vi "Begin.vi"(11 "Image Size":T1=enum."160x120") -> (0 "error out":errorcluster)   [LabVIEW 2012]
doc: "Called before other user functions, this VI is expected to open initial I/O refnums, load in file data, and do all program initialization. Notice that the <B>error out</B> terminal is simply used for data flow. Wiring it to other structures or subVIs ensures that this VI runs first."
uses:
  <vilib>/Rock Robotics/WPI/Camera/WPI_CameraImageSize.ctl
  <vilib>/Rock Robotics/WPI/Camera/WPI_CameraWhite Balance Values.ctl
  <vilib>/Rock Robotics/WPI/Camera/WPI_CameraExposure Values.ctl
  <vilib>/Rock Robotics/WPI/Camera/WPI_CameraFrameRate.ctl
  <vilib>/Rock Robotics/WPI/DriverStation/WPI_DriverStationRobotMode2.ctl
  <vilib>/Rock Robotics/SystemInterfaces/DIO/FPGA_DIOPWMChannel.ctl
  <vilib>/Rock Robotics/WPI/Joystick/WPI_JoystickDeviceEnum.ctl
  <vilib>/Rock Robotics/SystemInterfaces/DIO/FPGA_DIOChannel.ctl
  <vilib>/Rock Robotics/SystemInterfaces/AI/FPGA_AIGyroChannel.ctl
  <vilib>/Rock Robotics/WPI/Relay/WPI_RelayDirection.ctl
  <vilib>/Rock Robotics/SystemInterfaces/DIO/FPGA_DIORelayChannel.ctl
  <vilib>/Rock Robotics/SystemInterfaces/Typedef/FPGA_TypedefDigitalModule.ctl
  <vilib>/Rock Robotics/SystemInterfaces/AI/FPGA_AIChannel.ctl
  Robot Global Data.vi
  <vilib>/Rock Robotics/WPI/MotorControl/WPI_MotorControlOpen Victor.vi
  <vilib>/Rock Robotics/WPI/MotorControl/WPI_MotorControlOpen Jaguar.vi
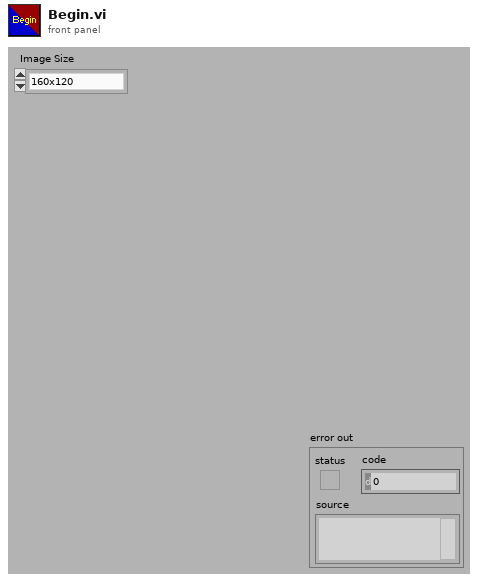
[diagram p1: front panel]
types:
  T1 = typedef "WPI_CameraImageSize.ctl" = enum16{"640x480", "320x240", "160x120"}
  T2 = typedef "FPGA_AIChannel.ctl" = enum8{"AI 1", "AI 2", "AI 3", "AI 4", "AI 5", "AI 6", "AI 7", "AI 8", "Invalid"}
  T3 = typedef "FPGA_DIOChannel.ctl" = enum8{"DIO 1", "DIO 2", "DIO 3", "DIO 4", "DIO 5", "DIO 6", "DIO 7", "DIO 8", "DIO 9", "DIO 10", "DIO 11", "DIO 12", "DIO 13", "DIO 14", "Invalid"}
  T4 = typedef "FPGA_TypedefDigitalModule.ctl" = enum16{"Digital Module 1", "Digital Module 2"}
  T5 = typedef "FPGA_DIOPWMChannel.ctl" = enum8{"PWM 1", "PWM 2", "PWM 3", "PWM 4", "PWM 5", "PWM 6", "PWM 7", "PWM 8", "PWM 9", "PWM 10", "Invalid"}
  T6 = typedef "FPGA_DIORelayChannel.ctl" = enum8{"Relay 1", "Relay 2", "Relay 3", "Relay 4", "Relay 5", "Relay 6", "Relay 7", "Relay 8", "Invalid"}
  T7 = typedef "WPI_RelayDirection.ctl" = enum16{"Both directions", "Forward only", "Reverse only"}
  T8 = typedef "FPGA_AIGyroChannel.ctl" = enum8{"AI 1", "AI 2", "Invalid"}
  T9 = typedef "WPI_JoystickDeviceEnum.ctl" = enum16{"USB 1", "USB 2", "USB 3", "USB 4", "Kinect 1", "Kinect 2"}
  T10 = typedef "WPI_DriverStationRobotMode2.ctl" = enum16{"Autonomous Disabled", "Autonomous Enabled", "Teleop Disabled", "Teleop Enabled", "Timeout", "Finish", "Test Disabled", "Test Enabled"}
  T11 = typedef "WPI_CameraFrameRate.ctl" = u32
  T12 = typedef "WPI_CameraExposure Values.ctl" = enum16{"Auto", "Flicker-free 50 Hz", "Flicker-free 60 Hz", "Hold current"}
  T13 = typedef "WPI_CameraWhite Balance Values.ctl" = enum16{"Auto", "Fixed indoor", "Fixed outdoor 1", "Fixed outdoor 2", "Fixed fluorescent 1", "Fixed fluorescent 2", "Hold current"}
  T14 = typedef "WPI_RelayDevRef.ctl" = cluster{"DevStatus":errorcluster, "Relay Channel":T6, "Digital Module":T4, "Relay Direction":T7}
  T15 = typedef "WPI_AnalogChannelDevRef.ctl" = cluster{"DevStatus":errorcluster, "Analog Module":T16, "Analog Channel":T2}
  T16 = typedef "FPGA_TypedefAnalogModule.ctl" = enum16{"Analog Module 1", "Analog Module 2"}
  T17 = typedef "WPI_DigitalInputDevRef.ctl" = cluster{"DevStatus":errorcluster, "DIO Channel":T3, "Digital Module":T4}
  T18 = typedef "WPI_CameraDevRef.ctl" = cluster{"Camera Address":string, "CameraStatus":errorcluster, "Acquire Image Notifier":refnum<notifier>}
  T19 = typedef "WPI_ServoDeviceRef.ctl" = cluster{"DeviceStatus":errorcluster, "Digital Module":T4, "PWM Channel":T5, "DeadBand":T20}
  T20 = typedef "WPI_PWMDeadband.ctl" = cluster{"Name":string, "maxPositivePwm":i32, "minPositivePwm":i32, "centerPwm":i32, "maxNegativePwm":i32, "minNegativePwm":i32, "angularRange":u16}
  T21 = typedef "WPI_MotorControlDeviceRef.ctl" = cluster{"DeviceStatus":errorcluster, "Type":enum16{"PWM", "CAN"}, "PWM":cluster{"Digital Module":T4, "PWM Channel":T5, "DeadBand":T20}, "CAN":cluster{"Device Number":u8, "Control Mode":T22, "Semaphore":T23, "Max Vout":dbl}, "Invert":bool, "TransformRef":T24, "InvTransformRef":T24}
  T22 = typedef "WPI_CANJaguar_ControlMode.ctl" = enum8{"Percent VBus", "Current", "Speed", "Position", "Voltage"}
  T23 = typedef "Semaphore RefNum" = refnum<k1>
  T24 = typedef "WPI_PWMTransform_ConPane.ctl" = refnum<vi>
  T25 = typedef "WPI_JoystickDevRef.ctl" = cluster{"Device":T9}
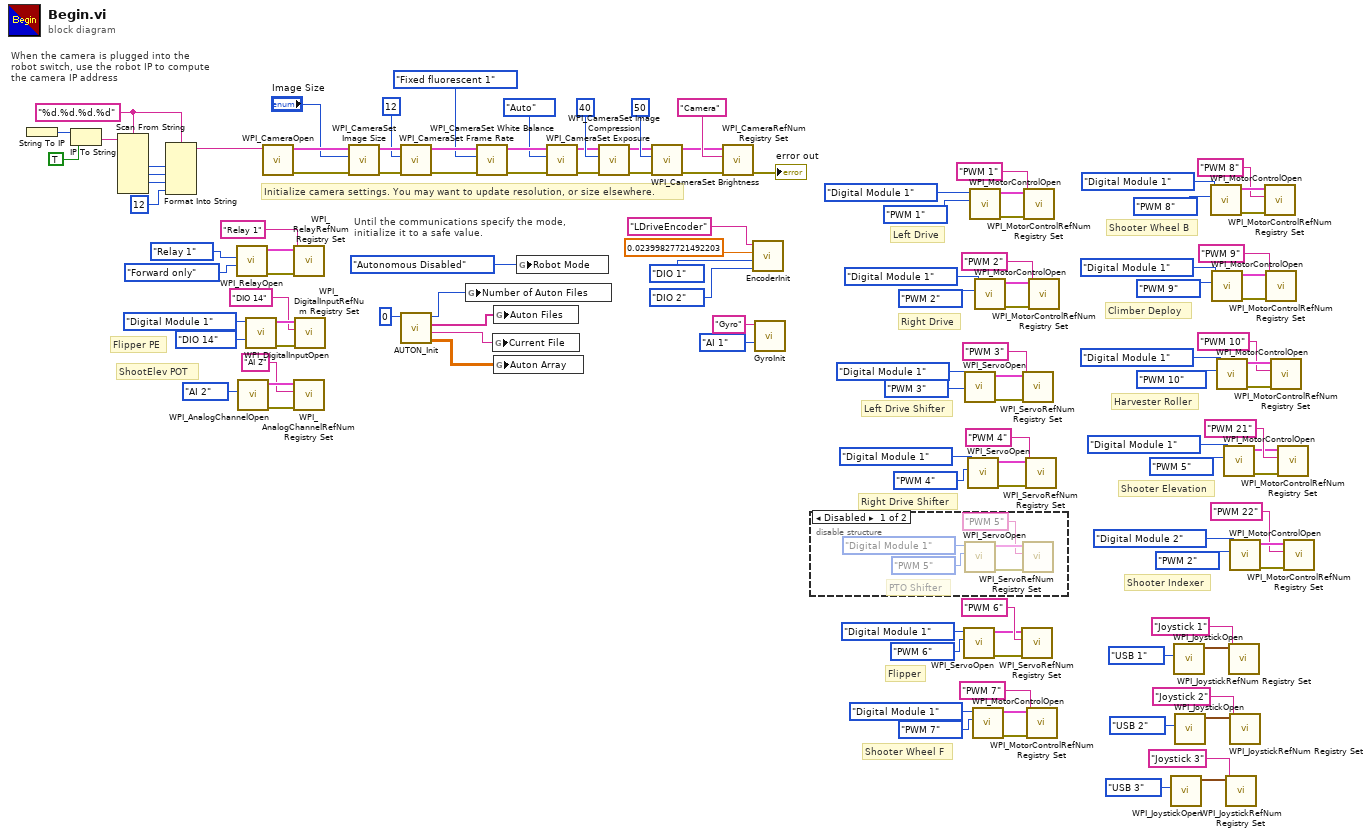
[diagram p0: block diagram]
diagram:
  w93 = "%d.%d.%d.%d" ("format string")
  # "ShootElev POT"
  # "Flipper PE"
  # "Flipper"
  # "Shooter Indexer"
  # "Shooter Elevation"
  # "Harvester Roller"
  # "Climber Deploy"
  # "Shooter Wheel B"
  # "Shooter Wheel F"
  # "Right Drive Shifter"
  # "Left Drive Shifter"
  # "Right Drive"
  # "Left Drive"
  # "Until the communications specify the mode,\ninitialize it to a safe value."
  # "When the camera is plugged into the\nrobot switch, use the robot IP to compute\nthe camera IP address"
  # "Initialize camera settings. You may want to update resolution, or size elsewhere."
  n1 = String To IP() -> (0:w100:u32)  [unwired: 1 in]
  n2 = IP To String(1:TRUE ("dot notation? (F)"), 2:w100) -> (0:w98:string)
  n3 = Scan From String(format string=w93, input string=w98) -> (output 1=w97:i32, output 2=w96:i32, output 3=w95:i32)  [unwired: 7 in, 3 out]
  n4 = Format Into String(format string=w93, w97, w96, w95, 12 ("Compression")) -> (resulting string=w91:string)  [unwired: 2 in, 1 out]
  n5 = call <vilib>:"WPI_RelayOpen.vi"("Relay Direction"=WPI_RelayDirection."Forward only", "Relay Channel"=FPGA_DIORelayChannel."Relay 1") -> ("error out"=w53:errorcluster, "RelayDevRef"=w52:T14)  [unwired: 8 in]
  n6 = call <vilib>:"WPI_AnalogChannelOpen.vi"("Analog Channel"=FPGA_AIChannel."AI 2") -> ("error out"=w4:errorcluster, "AIDeviceRef"=w3:T15)  [unwired: 9 in]
  n7 = call <vilib>:"WPI_DigitalInputOpen.vi"("DIO Channel"=FPGA_DIOChannel."DIO 14", "Digital Module (Module 1)"=FPGA_TypedefDigitalModule."Digital Module 1") -> ("error out"=w9:errorcluster, "DigitalInputDevRef"=w8:T17)  [unwired: 8 in]
  n8 = call <vilib>:"WPI_CameraOpen.vi"("Camera Address"=w91) -> ("error out"=w112:errorcluster, "CameraDevRef"=w113:T18)  [unwired: 1 in, 8 out]
  n9 = call <vilib>:"WPI_RelayRefNum Registry Set.vi"("error in (no error)"=w53, "refnum name"="Relay 1", "RelayDevRef"=w52) -> ()  [unwired: 7 in, 2 out]
  n10 = call <vilib>:"WPI_AnalogChannelRefNum Registry Set.vi"("error in (no error)"=w4, "refnum name"="AI 2", "AIDeviceRef"=w3) -> ()  [unwired: 7 in, 2 out]
  n11 = call <vilib>:"WPI_DigitalInputRefNum Registry Set.vi"("error in (no error)"=w9, "refnum name"="DIO 14", "DigitalInputDevRef"=w8) -> ()  [unwired: 7 in, 2 out]
  n12 = call <vilib>:"WPI_CameraSet Image Size.vi"("error in (no error)"=w112, "Image Size"="Image Size", "CameraDevRef"=w113) -> ("error out"=w111:errorcluster, "CameraDevRef Out"=w114:T18)  [unwired: 7 out]
  n13 = call <vilib>:"WPI_CameraSet Frame Rate.vi"("error in (no error)"=w111, "Frame Rate (fps)"=T11 12, "CameraDevRef"=w114) -> ("error out"=w110:errorcluster, "CameraDevRef Out"=w116:T18)  [unwired: 7 out]
  n14 = call "AUTON_Init.vi"("Default File"=0) -> ("Auton Array"=w60:dbl[][], "Current File"=w61:string, "Auton Files"=w62:string[], "Number of Auton Files"=w63:i64)  [unwired: 7 in]
  n15 = global write "Robot Global Data.vi" "Number of Auton Files"(w63) -> ()
  n16 = call <vilib>:"WPI_CameraSet White Balance.vi"("error in (no error)"=w110, "White Balance"=WPI_CameraWhite_Balance_Values."Fixed fluorescent 1", "CameraDevRef"=w116) -> ("error out"=w109:errorcluster, "CameraDevRef Out"=w115:T18)  [unwired: 7 out]
  n17 = global write "Robot Global Data.vi" "Current File"(w61) -> ()
  n18 = global write "Robot Global Data.vi" "Auton Files"(w62) -> ()
  n19 = global write "Robot Global Data.vi" "Auton Array"(w60) -> ()
  n20 = global write "Robot Global Data.vi" "Robot Mode"(WPI_DriverStationRobotMode2."Autonomous Disabled" ("Robot Mode")) -> ()
  n21 = call <vilib>:"WPI_CameraSet Exposure.vi"("error in (no error)"=w109, "Exposure"=WPI_CameraExposure_Values."Auto", "CameraDevRef"=w115) -> ("error out"=w108:errorcluster, "CameraDevRef Out"=w118:T18)  [unwired: 7 out]
  n22 = call <vilib>:"WPI_CameraSet Image Compression.vi"("error in (no error)"=w108, "Compression"=40, "CameraDevRef"=w118) -> ("error out"=w107:errorcluster, "CameraDevRef Out"=w117:T18)  [unwired: 7 out]
  n23 = call <vilib>:"WPI_CameraSet Brightness.vi"("error in (no error)"=w107, "Brightness"=50, "CameraDevRef"=w117) -> ("error out"=w105:errorcluster, "CameraDevRef Out"=w106:T18)  [unwired: 7 out]
  n24 = call <vilib>:"WPI_CameraRefNum Registry Set.vi"("error in (no error)"=w105, "refnum name"="Camera", "CameraDevRef"=w106) -> ("error out"=→"error out":errorcluster)  [unwired: 8 out]
  n25 = call "EncoderInit.vi"("refnum name"="LDriveEncoder", "DistancePerCount"=0.02399827721492203, "DIO Channel"=FPGA_DIOChannel."DIO 1", "DIO Channel 2"=FPGA_DIOChannel."DIO 2") -> ()  [unwired: 7 in]
  n26 = call "GyroInit.vi"("refnum name"="Gyro", "Analog Channel"=FPGA_AIGyroChannel."AI 1") -> ()  [unwired: 8 in]
  n27 = disable-structure shown="Disabled" {
    frame Disabled {
      # "PTO Shifter"
      n28 = call <vilib>:"WPI_ServoOpen.vi"("PWM Channel"=FPGA_DIOPWMChannel."PWM 5", "Digital Module (Module 1)"=FPGA_TypedefDigitalModule."Digital Module 1") -> ("error out"=w126:errorcluster, "ServoDeviceRef"=w125:T19)  [unwired: 8 in]
      n29 = call <vilib>:"WPI_ServoRefNum Registry Set.vi"("error in (no error)"=w126, "refnum name"="PWM 5", "ServoDeviceRef"=w125) -> ()  [unwired: 7 in, 2 out]
    }
    frame Enabled {
    }
  }
  n30 = call <vilib>:"WPI_ServoOpen.vi"("PWM Channel"=FPGA_DIOPWMChannel."PWM 6", "Digital Module (Module 1)"=FPGA_TypedefDigitalModule."Digital Module 1") -> ("error out"=w10:errorcluster, "ServoDeviceRef"=w11:T19)  [unwired: 8 in]
  n31 = call <vilib>:"WPI_ServoOpen.vi"("PWM Channel"=FPGA_DIOPWMChannel."PWM 3", "Digital Module (Module 1)"=FPGA_TypedefDigitalModule."Digital Module 1") -> ("error out"=w81:errorcluster, "ServoDeviceRef"=w80:T19)  [unwired: 8 in]
  n32 = call <vilib>:"WPI_ServoOpen.vi"("PWM Channel"=FPGA_DIOPWMChannel."PWM 4", "Digital Module (Module 1)"=FPGA_TypedefDigitalModule."Digital Module 1") -> ("error out"=w74:errorcluster, "ServoDeviceRef"=w75:T19)  [unwired: 8 in]
  n33 = call-poly <vilib>:"WPI_MotorControlOpen.vi"("PWM Channel"=FPGA_DIOPWMChannel."PWM 1", "Digital Module (Module 1)"=FPGA_TypedefDigitalModule."Digital Module 1") -> ("error out"=w89:errorcluster, "MotorControlDeviceRef"=w88:T21)  [unwired: 8 in]
  n34 = call-poly <vilib>:"WPI_MotorControlOpen.vi"("PWM Channel"=FPGA_DIOPWMChannel."PWM 7", "Digital Module (Module 1)"=FPGA_TypedefDigitalModule."Digital Module 1") -> ("error out"=w45:errorcluster, "MotorControlDeviceRef"=w46:T21)  [unwired: 8 in]
  n35 = call-poly <vilib>:"WPI_MotorControlOpen.vi"("PWM Channel"=FPGA_DIOPWMChannel."PWM 2", "Digital Module (Module 1)"=FPGA_TypedefDigitalModule."Digital Module 1") -> ("error out"=w82:errorcluster, "MotorControlDeviceRef"=w83:T21)  [unwired: 8 in]
  n36 = call <vilib>:"WPI_ServoRefNum Registry Set.vi"("error in (no error)"=w10, "refnum name"="PWM 6", "ServoDeviceRef"=w11) -> ()  [unwired: 7 in, 2 out]
  n37 = call <vilib>:"WPI_ServoRefNum Registry Set.vi"("error in (no error)"=w81, "refnum name"="PWM 3", "ServoDeviceRef"=w80) -> ()  [unwired: 7 in, 2 out]
  n38 = call <vilib>:"WPI_MotorControlRefNum Registry Set.vi"("error in (no error)"=w89, "refnum name"="PWM 1", "MotorControlDevRef"=w88) -> ()  [unwired: 7 in, 2 out]
  n39 = call <vilib>:"WPI_ServoRefNum Registry Set.vi"("error in (no error)"=w74, "refnum name"="PWM 4", "ServoDeviceRef"=w75) -> ()  [unwired: 7 in, 2 out]
  n40 = call <vilib>:"WPI_MotorControlRefNum Registry Set.vi"("error in (no error)"=w45, "refnum name"="PWM 7", "MotorControlDevRef"=w46) -> ()  [unwired: 7 in, 2 out]
  n41 = call <vilib>:"WPI_MotorControlRefNum Registry Set.vi"("error in (no error)"=w82, "refnum name"="PWM 2", "MotorControlDevRef"=w83) -> ()  [unwired: 7 in, 2 out]
  n42 = call <vilib>:"WPI_JoystickOpen.vi"("JoystickDevice"=WPI_JoystickDeviceEnum."USB 3") -> ("JoystickDevRef"=w67:T25)  [unwired: 10 in]
  n43 = call <vilib>:"WPI_JoystickOpen.vi"("JoystickDevice"=WPI_JoystickDeviceEnum."USB 1") -> ("JoystickDevRef"=w73:T25)  [unwired: 10 in]
  n44 = call <vilib>:"WPI_JoystickOpen.vi"("JoystickDevice"=WPI_JoystickDeviceEnum."USB 2") -> ("JoystickDevRef"=w68:T25)  [unwired: 10 in]
  n45 = call-poly <vilib>:"WPI_MotorControlOpen.vi"("PWM Channel"=FPGA_DIOPWMChannel."PWM 8", "Digital Module (Module 1)"=FPGA_TypedefDigitalModule."Digital Module 1") -> ("error out"=w38:errorcluster, "MotorControlDeviceRef"=w39:T21)  [unwired: 8 in]
  n46 = call-poly <vilib>:"WPI_MotorControlOpen.vi"("PWM Channel"=FPGA_DIOPWMChannel."PWM 9", "Digital Module (Module 1)"=FPGA_TypedefDigitalModule."Digital Module 1") -> ("error out"=w44:errorcluster, "MotorControlDeviceRef"=w43:T21)  [unwired: 8 in]
  n47 = call-poly <vilib>:"WPI_MotorControlOpen.vi"("PWM Channel"=FPGA_DIOPWMChannel."PWM 10", "Digital Module (Module 1)"=FPGA_TypedefDigitalModule."Digital Module 1") -> ("error out"=w34:errorcluster, "MotorControlDeviceRef"=w35:T21)  [unwired: 8 in]
  n48 = call-poly <vilib>:"WPI_MotorControlOpen.vi"("PWM Channel"=FPGA_DIOPWMChannel."PWM 5", "Digital Module (Module 1)"=FPGA_TypedefDigitalModule."Digital Module 1") -> ("error out"=w22:errorcluster, "MotorControlDeviceRef"=w21:T21)  [unwired: 8 in]
  n49 = call <vilib>:"WPI_JoystickRefNum Registry Set.vi"("refnum name"="Joystick 3", "JoystickDevRef"=w67) -> ()  [unwired: 8 in, 2 out]
  n50 = call <vilib>:"WPI_JoystickRefNum Registry Set.vi"("refnum name"="Joystick 1", "JoystickDevRef"=w73) -> ()  [unwired: 8 in, 2 out]
  n51 = call-poly <vilib>:"WPI_MotorControlOpen.vi"("PWM Channel"=FPGA_DIOPWMChannel."PWM 2", "Digital Module (Module 1)"=FPGA_TypedefDigitalModule."Digital Module 2") -> ("error out"=w17:errorcluster, "MotorControlDeviceRef"=w18:T21)  [unwired: 8 in]
  n52 = call <vilib>:"WPI_JoystickRefNum Registry Set.vi"("refnum name"="Joystick 2", "JoystickDevRef"=w68) -> ()  [unwired: 8 in, 2 out]
  n53 = call <vilib>:"WPI_MotorControlRefNum Registry Set.vi"("error in (no error)"=w38, "refnum name"="PWM 8", "MotorControlDevRef"=w39) -> ()  [unwired: 7 in, 2 out]
  n54 = call <vilib>:"WPI_MotorControlRefNum Registry Set.vi"("error in (no error)"=w44, "refnum name"="PWM 9", "MotorControlDevRef"=w43) -> ()  [unwired: 7 in, 2 out]
  n55 = call <vilib>:"WPI_MotorControlRefNum Registry Set.vi"("error in (no error)"=w34, "refnum name"="PWM 10", "MotorControlDevRef"=w35) -> ()  [unwired: 7 in, 2 out]
  n56 = call <vilib>:"WPI_MotorControlRefNum Registry Set.vi"("error in (no error)"=w22, "refnum name"="PWM 21", "MotorControlDevRef"=w21) -> ()  [unwired: 7 in, 2 out]
  n57 = call <vilib>:"WPI_MotorControlRefNum Registry Set.vi"("error in (no error)"=w17, "refnum name"="PWM 22", "MotorControlDevRef"=w18) -> ()  [unwired: 7 in, 2 out]
